vi "Fetch_Item.vi"(8 "error in (no error)":errorcluster, 11 "itemID":string) -> (0 "error out":errorcluster, 2 "index":i32, 3 "IB_Tree_Item_Proj out":refnum<class "IB_Tree_Item_Proj.lvclass">)   [LabVIEW 2020, in "IB_Tree_Item_Proj.lvclass"]
uses:
  <vilib>/AppBuilder/IB_Classes/Tree_Item_Proj/IB_Tree_Item_Proj.lvclass
  <vilib>/AppBuilder/IB_Classes/Tree_Item_Proj/IB_Tree_Item_Proj.lvclass/IB_Tree_Item_Proj.ctl
  <vilib>/AppBuilder/IB_Classes/Tree_Item/IB_Tree_Item.lvclass
  e:/builds/penguin/labview/branches/2020/dev/dist/vi.lib/AppBuilder/IB_Classes/Tree_Item/IB_Tree_Item.lvclass
  e:/builds/penguin/labview/branches/2020/dev/dist/vi.lib/AppBuilder/IB_Classes/Tree_Item_Proj/IB_Tree_Item_Proj.lvclass
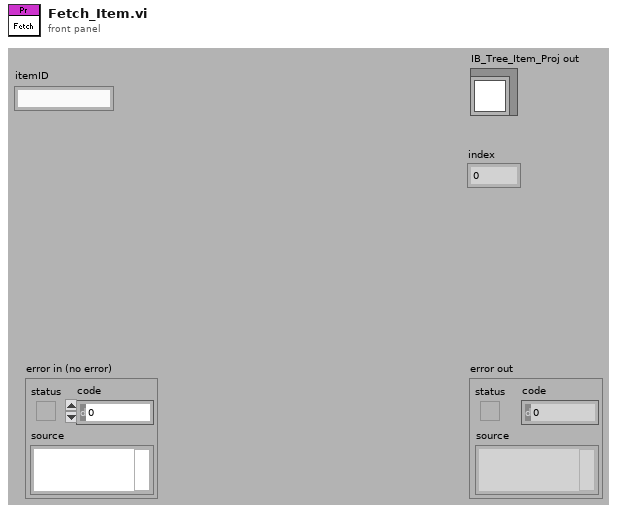
[diagram p1: front panel]
types:
  T1 = typedef "IB_Tree_Item.ctl" = cluster{"symbol index":i32, "child tag":string, "parentTag":string, "left cell name":string}
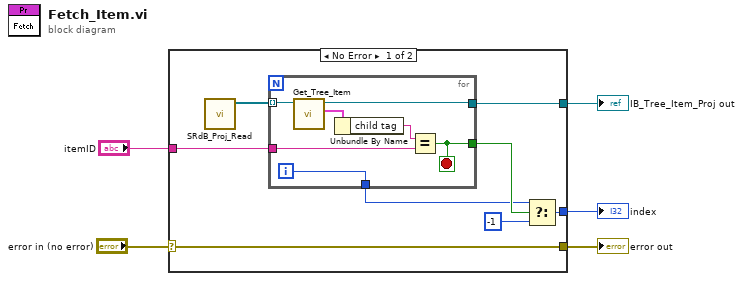
[diagram p0: block diagram]
diagram:
  n1 = case shown="No Error" "error in (no error)" {
    selector: "error in (no error)" -> [w13 w21]
    tunnel: [w13 w21] -> w4
    tunnel: [w11 _] -> w3
    tunnel: "itemID" -> [w12 _]
    tunnel: [w6 _] -> w1
    frame No Error {
      n2 = call <resource>:"SRdB_Proj_Read.vi"() -> ("Proj Items"=w10:refnum<class "IB_Tree_Item_Proj.lvclass">[])  [unwired: 10 in, 1 out]
      n3 = for {
        tunnel: w10 -> [w16] mode=indexing
        tunnel: w12 -> [w19]
        tunnel: [w15] -> w11
        tunnel: [w18] -> w9
        tunnel: [w17] -> w8
        i -> [w17]
        stop <- w18 stop-if-true
        n4 = call <vilib>:"Get_Tree_Item.vi"("IB_TreeItem in"=w16) -> ("data"=w14:T1, "IB_TreeItem out"=w15:refnum<class "IB_Tree_Item_Proj.lvclass">)  [unwired: 8 in, 1 out]
        n5 = Unbundle By Name(w14) -> ("child tag"=w20:string)
        n6 = Equal?(x=w20, y=w19) -> (x = y?=w18:bool)
      }
      n7 = Select(t=w8, s=w9, f=-1) -> (s? t:f=w6:i32)
    }
    frame Error {
    }
  }
  "error out" <- w4
  "IB_Tree_Item_Proj out" <- w3
  "index" <- w1
